vi "_JKISMQFGV.vi"(6 "?":T3, 8 "Error in":errorcluster caption="Error in (no error)", 9 "create if not found? (T)":bool=TRUE, 11 "Name(\"\" to use uuid) in":string) -> (0 "Error out":errorcluster, 1 "Boolean":bool, 2 "Name":string[](array[string]), 3 "Array":T1[](array[typedef]))   [LabVIEW 2014, in "JKI-State-Machine-Plus.lvlib"]
uses:
  JKI-State-Machine-Plus.lvlib
  _JKISMQFGVOPER.ctl
  _JKISMQ.ctl
  Typedef/_Cross JKI StateMachine State Data.ctl
  Typedef/_JKISM_MSG_TYPE.ctl
  Typedef/_Cross JKI StateMachine State Response.ctl
  Typedef/_JKISM_MODE.ctl
  FGV-BroadcastRegistry/Oper-BroadcastRegistry.ctl
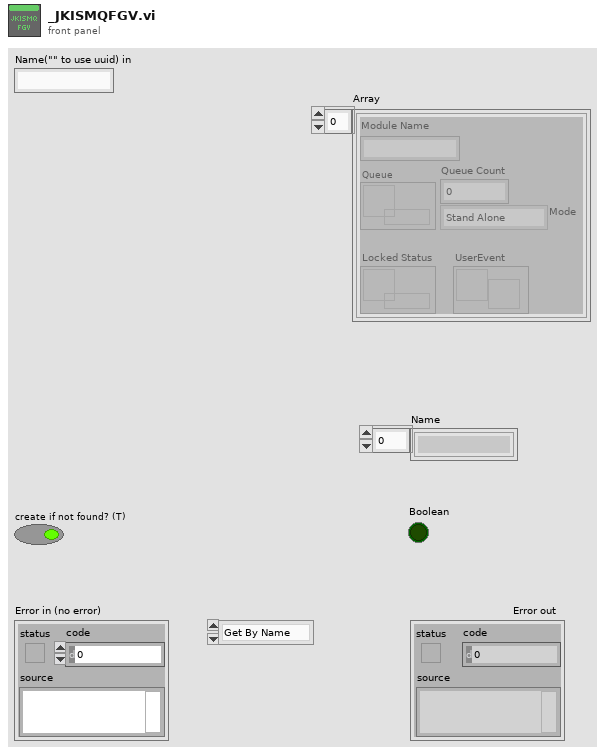
[diagram p1: front panel]
types:
  T1 = typedef "JKI-State-Machine-Plus.lvlib/_JKISMQ.ctl" = cluster{"Module Name":string, "Queue":refnum<queue>, "Locked Status":refnum<data-value>, "Mode":T2, "UserEvent":refnum<user-event>, "Queue Count":i32}
  T2 = typedef "JKI-State-Machine-Plus.lvlib/_JKISM_MODE.ctl" = enum16{"Stand Alone", "JKISM", "Action Worker"}
  T3 = typedef "JKI-State-Machine-Plus.lvlib/_JKISMQFGVOPER.ctl" = enum16{"Get By Name", "List", "Check If Name Exists", "Release", "Module Status"}
  T4 = typedef "JKI-State-Machine-Plus.lvlib/Oper-BroadcastRegistry.ctl" = enum16{"Delete Source Module", "Delete Dest Module", "Remove Module", "Register", "Unregister", "Check"}
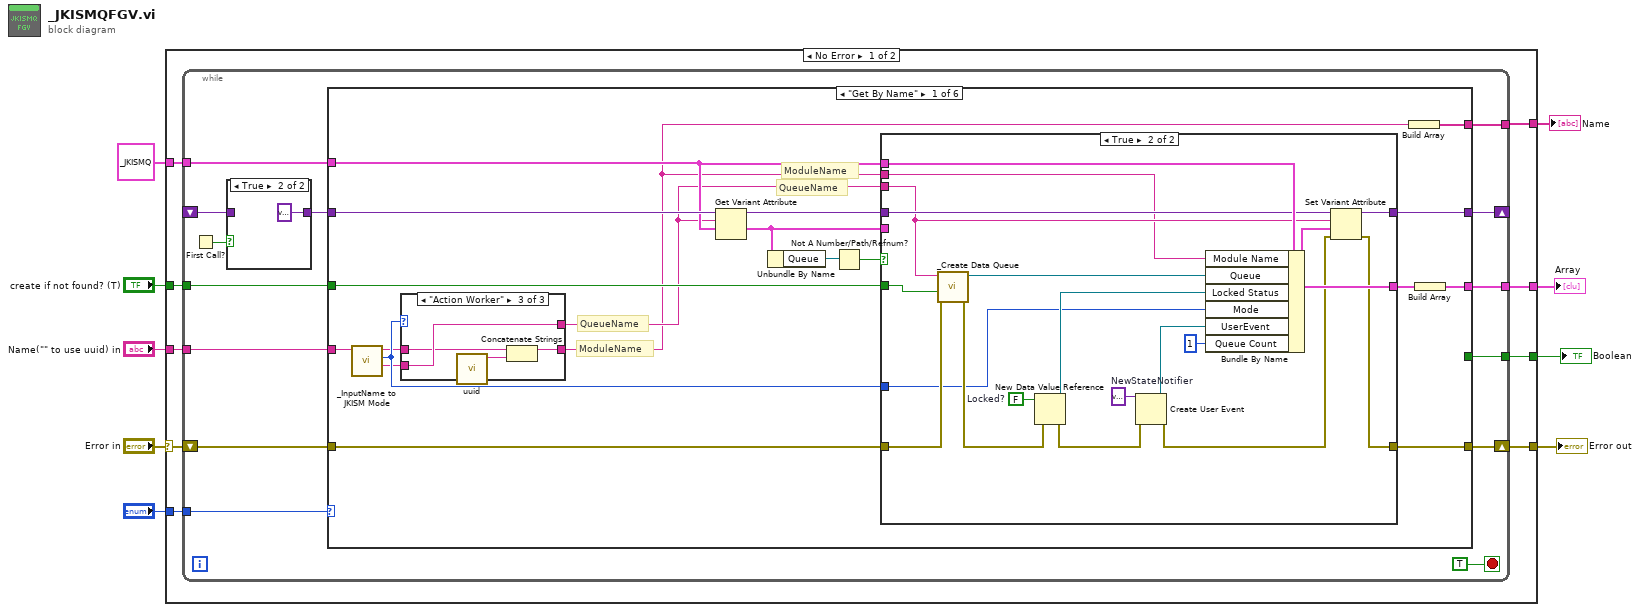
[diagram p0: block diagram]
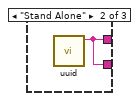
[diagram p4: hidden frame]
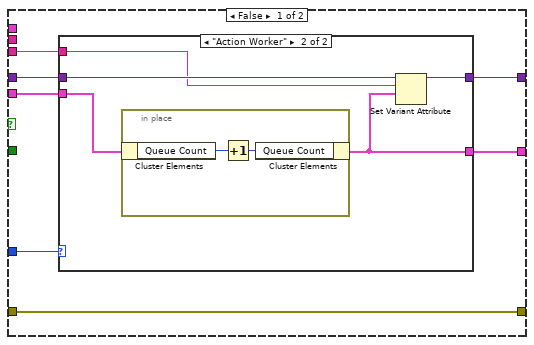
[diagram p5: hidden frame]
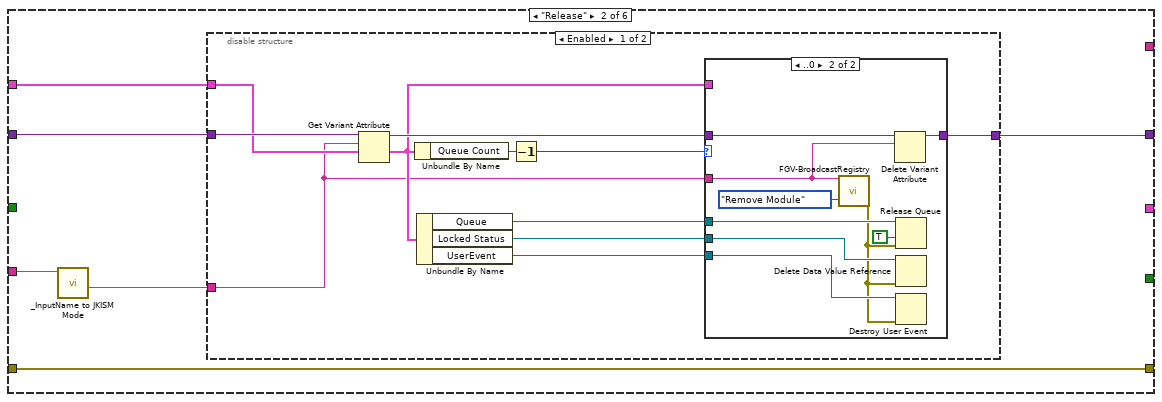
[diagram p7: hidden frame]
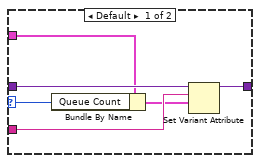
[diagram p8: hidden frame]
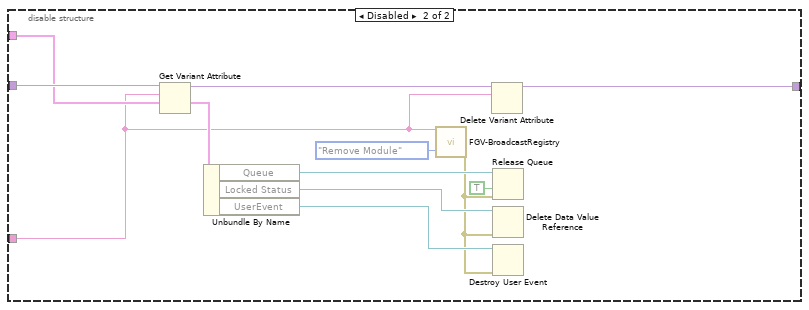
[diagram p9: hidden frame]
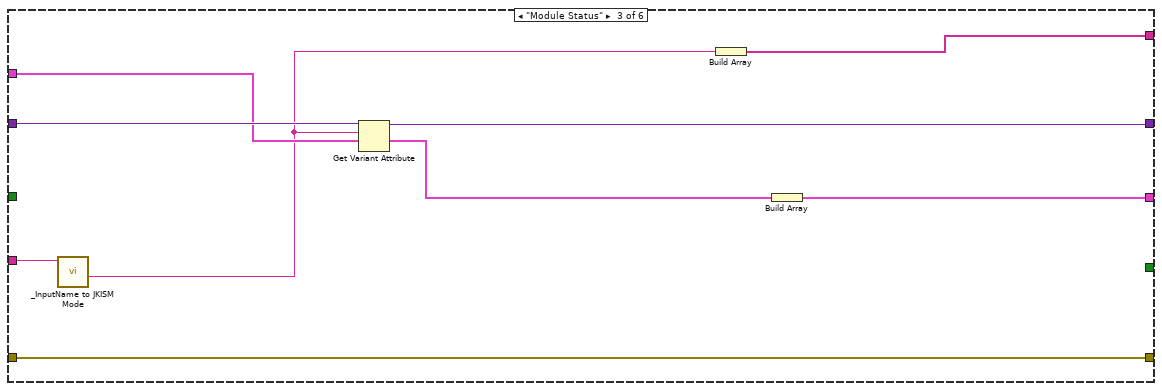
[diagram p10: hidden frame]
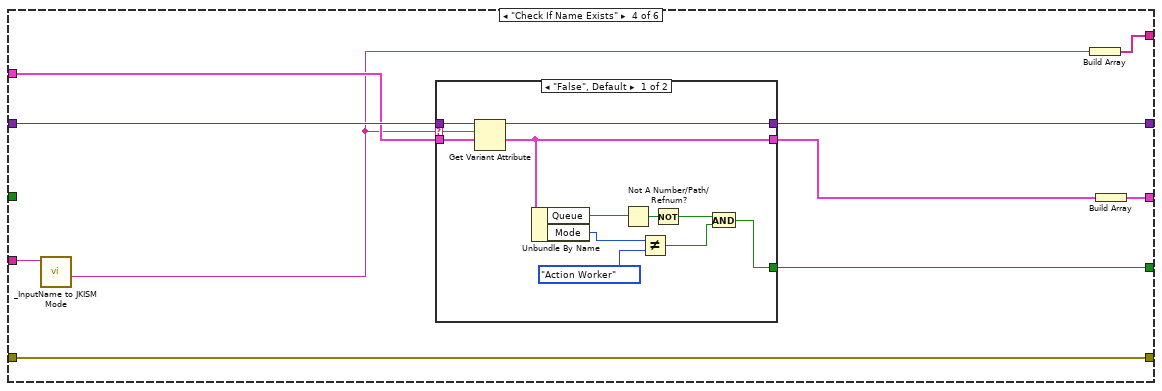
[diagram p11: hidden frame]
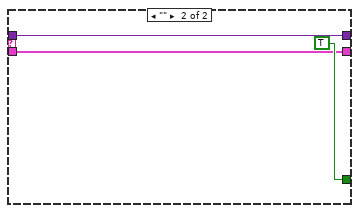
[diagram p12: hidden frame]
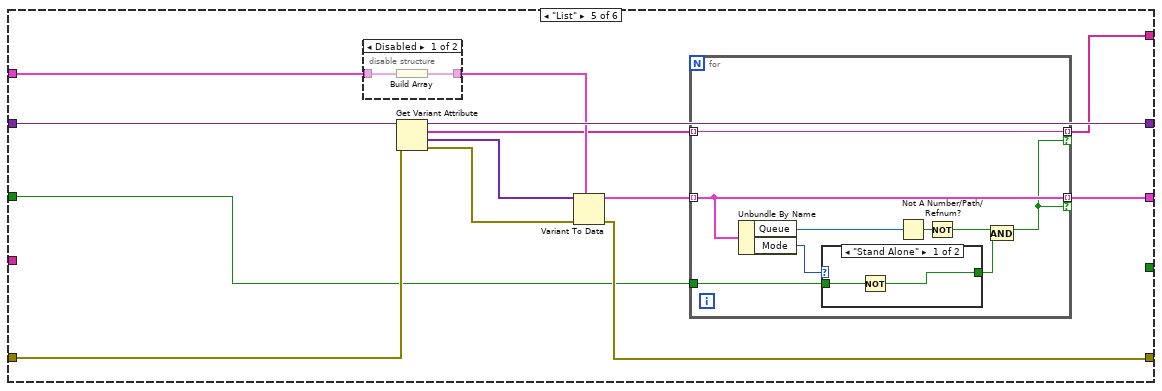
[diagram p13: hidden frame]
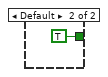
[diagram p14: hidden frame]
diagram:
  n1 = case shown="No Error" "Error in" {
    selector: "Error in" -> [w15 w202]
    tunnel: "?" -> [w18 _]
    tunnel: "Name(\"\" to use uuid) in" -> [w17 _]
    tunnel: "create if not found? (T)" -> [w16 _]
    tunnel: [w14 w202] -> w5
    tunnel: [w13 _] -> w4
    tunnel: T1 {"Module Name"="", "Queue"=refnum, "Locked Status"=refnum, "Mode"=enum."Stand Alone", "UserEvent"=refnum, "Queue Count"=0} ("JKISMQ") -> [w12 _]
    tunnel: [w11 _] -> w2
    tunnel: [w10 _] -> w1
    frame No Error {
      n2 = while {
        tunnel: w18 -> [w31]
        tunnel: w17 -> [w30]
        tunnel: w16 -> [w29]
        tunnel: [w28] -> w11
        shift-right: [w24] -> _
        shift-left: _ -> [w26]
        shift-right: [w22] -> w14
        shift-left: w15 -> [w23]
        tunnel: [w21] -> w13
        tunnel: w12 -> [w20]
        tunnel: [w19] -> w10
        stop <- TRUE stop-if-true
        n3 = First Call?() -> (First Call?: T/F=w27:bool)
        n4 = case shown="True" w27 {
          tunnel: [w33 variant] -> w25
          tunnel: w26 -> [w33 _]
          frame False {
          }
          frame True {
          }
        }
        n5 = case shown="\"Get By Name\"" w31 {
          tunnel: w30 -> [w40 w96 w144 w149 _ _]
          tunnel: w29 -> [w53 _ _ _ w173 _]
          tunnel: [w42 _ w141 w152 w177 _] -> w28
          tunnel: w25 -> [w51 w99 w146 w157 w185 w201]
          tunnel: [w49 w98 w143 w156 w184 w201] -> w24
          tunnel: w23 -> [w45 w100 w147 w154 w175 w200]
          tunnel: [w44 w100 w147 w154 w174 w200] -> w22
          tunnel: [w41 _ w139 w151 w178 _] -> w21
          tunnel: w20 -> [w43 w97 w145 w153 w182 _]
          tunnel: [_ _ _ w150 _ _] -> w19
          frame "Get By Name" {
            # "ModuleName"
            # "QueueName"
            # "ModuleName"
            # "QueueName"
            n6 = call "_InputName to JKISM Mode.vi"("String"=w40) -> ("QName"=w37:string, "JKISM Mode"=w39:T2, "String(dup)"=w38:string)  [unwired: 8 in]
            n7 = case shown="\"Action Worker\"" w39 {
              tunnel: [w54 w55 w59] -> w36
              tunnel: [w54 w55 w56] -> w35
              tunnel: w38 -> [w54 _ w58]
              tunnel: w37 -> [_ _ w59]
              frame "JKISM" {
              }
              frame "Stand Alone" {
                n8 = call "uuid.vi"() -> ("UUID"=w55:string)  [unwired: 11 in]
              }
              frame "Action Worker" {
                n9 = call "uuid.vi"() -> ("UUID"=w57:string)  [unwired: 11 in]
                n10 = Concatenate Strings(w58, w57) -> (w56:string)
              }
            }
            n11 = Get Variant Attribute(Variant=w51, name=w36, default value (empty Variant)=w43) -> (duplicate Variant=w50:variant, value=w48:T1)  [unwired: 1 in, 2 out]
            n12 = Unbundle By Name(w48) -> ("Queue"=w47:refnum<queue>)
            n13 = Not A Number/Path/Refnum?(number/path/refnum=w47) -> (NaN/Path/Refnum?=w46:bool)
            n14 = case shown="True" w46 {
              tunnel: w53 -> [_ w93]
              tunnel: [w62 w87] -> w52
              tunnel: w36 -> [w60 w77]
              tunnel: w43 -> [_ w90]
              tunnel: w50 -> [w63 w89]
              tunnel: [w64 w88] -> w49
              tunnel: w48 -> [w61 _]
              tunnel: w45 -> [w66 w86]
              tunnel: [w66 w84] -> w44
              tunnel: w39 -> [w65 w79]
              tunnel: w35 -> [_ w76]
              frame False {
                n15 = case shown="\"Action Worker\"" w65 {
                  tunnel: [w68 w72] -> w64
                  tunnel: w63 -> [w68 w73]
                  tunnel: [w67 w69] -> w62
                  tunnel: w61 -> [w67 w70]
                  tunnel: w60 -> [_ w71]
                  frame Default {
                  }
                  frame "Action Worker" {
                    n16 = in-place {
                      n17 = in-place-cluster #1(w70) -> ("Queue Count"=w75:i32)
                      n18 = Increment(x=w75) -> (x+1=w74:i32)
                      n19 = in-place-cluster #1("Queue Count"=w74) -> (w69:T1)
                    }
                    n20 = Set Variant Attribute(Variant=w73, name=w71, value=w69) -> (Variant out=w72:variant)  [unwired: 1 in, 2 out]
                  }
                }
              }
              frame True {
                w83 = variant  # NewStateNotifier
                w94 = FALSE  # Locked?
                n21 = call "_Create Data Queue.vi"("error in (no error)"=w86, "create if not found? (T)"=w93, "Name"=w77) -> ("error out"=w85:errorcluster, "Queue out"=w92:refnum<queue>)  [unwired: 6 in, 1 out]
                n22 = New Data Value Reference(data value=w94, error in=w85) -> (data value reference=w91:refnum<data-value>, error out=w82:errorcluster)
                n23 = Create User Event(user event datatype=w83, error in=w82) -> (user event=w81:refnum<user-event>, error out=w80:errorcluster)
                n24 = Bundle By Name(cluster=w90, "Module Name"=w76, "Queue"=w92, "Locked Status"=w91, "Mode"=w79, "UserEvent"=w81, "Queue Count"=1) -> (w87:T1)
                n25 = Set Variant Attribute(Variant=w89, name=w77, value=w87, error in=w80) -> (Variant out=w88:variant, error out=w84:errorcluster)  [unwired: 1 out]
              }
            }
            n26 = Build Array(w35) -> (w41:string[])
            n27 = Build Array(w52) -> (w42:T1[])
          }
          frame "Release" {
            n28 = call "_InputName to JKISM Mode.vi"("String"=w96) -> ("QName"=w95:string)  [unwired: 8 in, 2 out]
            n29 = disable-structure shown="Enabled" {
              disable-tunnel: w99 -> [w108 w135]
              disable-tunnel: [w104 w133] -> w98
              disable-tunnel: w97 -> [w103 w132]
              disable-tunnel: w95 -> [w101 w130]
              frame Enabled {
                n30 = Get Variant Attribute(Variant=w108, name=w101, default value (empty Variant)=w103) -> (duplicate Variant=w105:variant, value=w102:T1)  [unwired: 1 in, 2 out]
                n31 = Unbundle By Name(w102) -> ("Queue Count"=w107:i32)
                n32 = Unbundle By Name(w102) -> ("Queue"=w111:refnum<queue>, "Locked Status"=w110:refnum<data-value>, "UserEvent"=w109:refnum<user-event>)
                n33 = Decrement(x=w107) -> (x-1=w106:i32)
                n34 = case shown="..0" w106 {
                  selector: w106 -> [w112 _]
                  tunnel: w111 -> [_ w126]
                  tunnel: w110 -> [_ w124]
                  tunnel: w109 -> [_ w123]
                  tunnel: w101 -> [w114 w118]
                  tunnel: w105 -> [w117 w120]
                  tunnel: [w116 w119] -> w104
                  tunnel: w102 -> [w115 _]
                  frame Default {
                    n35 = Bundle By Name(cluster=w115, "Queue Count"=w112) -> (w113:T1)
                    n36 = Set Variant Attribute(Variant=w117, name=w114, value=w113) -> (Variant out=w116:variant)  [unwired: 1 in, 2 out]
                  }
                  frame ..0 {
                    n37 = call "FGV-BroadcastRegistry.vi"("Source"=w118, "Operation"=Oper-BroadcastRegistry."Remove Module") -> ("Error out"=w121:errorcluster)  [unwired: 11 in, 2 out]
                    n38 = Delete Variant Attribute(6:w118, 7:w120) -> (3:w119:variant)  [unwired: 1 in, 2 out]
                    n39 = Release Queue(queue=w126, force destroy? (F)=TRUE, error in (no error)=w121) -> ()  [unwired: 3 out]
                    n40 = Delete Data Value Reference(data value reference=w124, error in=w121) -> ()  [unwired: 2 out]
                    n41 = Destroy User Event(user event=w123, error in=w121) -> ()  [unwired: 1 out]
                  }
                }
              }
              frame Disabled {
                n42 = Get Variant Attribute(Variant=w135, name=w130, default value (empty Variant)=w132) -> (duplicate Variant=w134:variant, value=w131:T1)  [unwired: 1 in, 2 out]
                n43 = Unbundle By Name(w131) -> ("Queue"=w138:refnum<queue>, "Locked Status"=w137:refnum<data-value>, "UserEvent"=w136:refnum<user-event>)
                n44 = call "FGV-BroadcastRegistry.vi"("Source"=w130, "Operation"=Oper-BroadcastRegistry."Remove Module") -> ("Error out"=w127:errorcluster)  [unwired: 11 in, 2 out]
                n45 = Delete Variant Attribute(6:w130, 7:w134) -> (3:w133:variant)  [unwired: 1 in, 2 out]
                n46 = Release Queue(queue=w138, force destroy? (F)=TRUE, error in (no error)=w127) -> ()  [unwired: 3 out]
                n47 = Delete Data Value Reference(data value reference=w137, error in=w127) -> ()  [unwired: 2 out]
                n48 = Destroy User Event(user event=w136, error in=w127) -> ()  [unwired: 1 out]
              }
            }
          }
          frame "Module Status" {
            n49 = call "_InputName to JKISM Mode.vi"("String"=w144) -> ("QName"=w140:string)  [unwired: 8 in, 2 out]
            n50 = Get Variant Attribute(Variant=w146, name=w140, default value (empty Variant)=w145) -> (duplicate Variant=w143:variant, value=w142:T1)  [unwired: 1 in, 2 out]
            n51 = Build Array(w140) -> (w139:string[])
            n52 = Build Array(w142) -> (w141:T1[])
          }
          frame "Check If Name Exists" {
            n53 = call "_InputName to JKISM Mode.vi"("String"=w149) -> ("QName"=w148:string)  [unwired: 8 in, 2 out]
            n54 = case shown="\"False\", Default" w148 {
              selector: w148 -> [w166 _]
              tunnel: w157 -> [w169 w172]
              tunnel: [w168 w172] -> w156
              tunnel: [w165 w170] -> w155
              tunnel: w153 -> [w167 w170]
              tunnel: [w161 TRUE] -> w150
              frame "False", Default {
                n55 = Get Variant Attribute(Variant=w169, name=w166, default value (empty Variant)=w167) -> (duplicate Variant=w168:variant, value=w165:T1)  [unwired: 1 in, 2 out]
                n56 = Unbundle By Name(w165) -> ("Queue"=w164:refnum<queue>, "Mode"=w160:T2)
                n57 = Not A Number/Path/Refnum?(number/path/refnum=w164) -> (NaN/Path/Refnum?=w163:bool)
                n58 = Not Equal?(x=w160, y=_JKISM_MODE."Action Worker") -> (x != y?=w158:bool)
                n59 = Not(x=w163) -> (.not. x?=w162:bool)
                n60 = And(x=w162, y=w158) -> (x .and. y?=w161:bool)
              }
              frame "" {
              }
            }
            n61 = Build Array(w148) -> (w151:string[])
            n62 = Build Array(w155) -> (w152:T1[])
          }
          frame "List" {
            n63 = disable-structure shown="Disabled" {
              disable-tunnel: w182 -> [w199 _]
              disable-tunnel: [w198 _] -> w181
              frame Disabled {
                n64 = Build Array(w199) -> (w198:T1[])
              }
              frame Enabled {
              }
            }
            n65 = Get Variant Attribute(Variant=w185, error in=w175) -> (duplicate Variant=w184:variant, names=w179:string[], values=w183:variant[], error out=w176:errorcluster)  [unwired: 2 in]
            n66 = Variant To Data(error in=w176, type=w181, Variant=w183) -> (data=w180:T1[], error out=w174:errorcluster)
            n67 = for {
              tunnel: w180 -> [w193] mode=indexing
              tunnel: w179 -> [w194] mode=indexing
              tunnel: [w194] -> w178 mode=indexing if=w190
              tunnel: [w193] -> w177 mode=indexing if=w190
              tunnel: w173 -> [w186]
              n68 = Unbundle By Name(w193) -> ("Queue"=w192:refnum<queue>, "Mode"=w188:T2)
              n69 = case shown="\"Stand Alone\"" w188 {
                tunnel: [w195 TRUE] -> w187
                tunnel: w186 -> [w196 _]
                frame "Stand Alone" {
                  n70 = Not(x=w196) -> (.not. x?=w195:bool)
                }
                frame Default {
                }
              }
              n71 = Not A Number/Path/Refnum?(number/path/refnum=w192) -> (NaN/Path/Refnum?=w191:bool)
              n72 = Not(x=w191) -> (.not. x?=w189:bool)
              n73 = And(x=w189, y=w187) -> (x .and. y?=w190:bool)
            }
          }
          frame Default {
          }
        }
      }
    }
    frame Error {
    }
  }
  "Error out" <- w5
  "Name" <- w4
  "Array" <- w2
  "Boolean" <- w1
